vi "Configure External Trigger.vi"(8 "error in (no error)":errorcluster {"code" format="%.0x"}, 9 "external trigger polarity (Positive)":i32(ring)=1 items=["Positive"=1, "Negative"=2], 10 "external trigger level":dbl, 11 "instrument handle":refnum<k15>) -> (0 "error out":errorcluster {"code" format="%.0x"}, 3 "instrument handle out":refnum<k15>)   [LabVIEW 2009, in "Keysight XSAn.lvlib"]
doc: "This VI specifies the external level and slope for triggering.\n\nSupported Models: All supported"
uses:
  <instrlib>/Keysight XSAn/Keysight XSAn.lvlib
  AgXSAn.dll
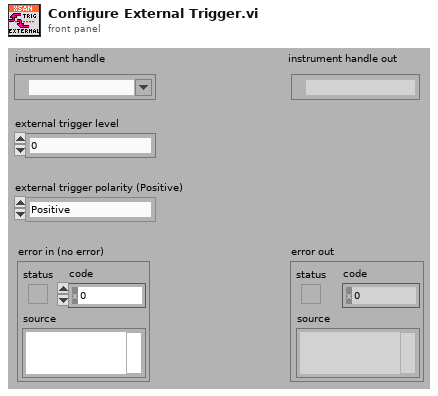
[diagram p1: front panel]
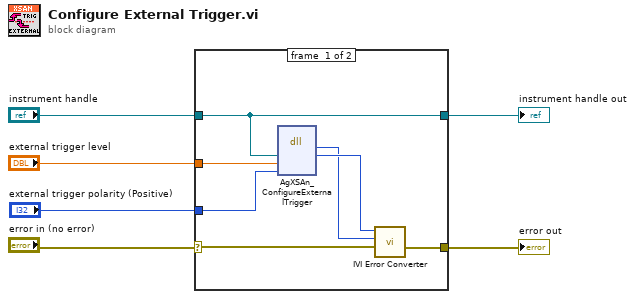
[diagram p0: block diagram]
diagram:
  n1 = case shown="No Error" "error in (no error)" {
    selector: "error in (no error)" -> [w11 w15]
    tunnel: [w12 w15] -> w5
    tunnel: "instrument handle" -> [w9 w14]
    tunnel: [w9 w14] -> w3
    tunnel: "external trigger polarity (Positive)" -> [w8 _]
    tunnel: "external trigger level" -> [w7 _]
    frame #0 {
      n2 = dll-call lib="AgXSAn**.dll" fn="AgXSAn_ConfigureExternalTrigger" ("LabVIEW:IviSpecAn_ConfigureExternalTrigger")("instrument handle"=w9, "external trigger level"=w7, "external trigger polarity"=w8) -> ("Status"=w10:i32, "instrument handle"=w13:u32)  [unwired: 5 in, 2 out]
      n3 = call <instrlib>:"IVI Error Converter.vi"("error in (no error)"=w11, "IVI error code (0)"=w10, "instrument handle"=w13) -> ("error out"=w12:errorcluster)  [unwired: 7 in, 1 out]
    }
    frame #1 {
    }
  }
  "error out" <- w5
  "instrument handle out" <- w3
